vi "Close Tab Button - Tab Width--Const.vi"() -> (3 "Tab Width":i32)   [LabVIEW 2017]
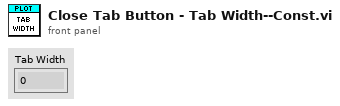
[diagram p1: front panel]
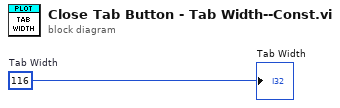
[diagram p0: block diagram]
diagram:
  w1 = 116  # Tab Width
  "Tab Width" <- w1
